vi "ServoAction.vi"(7 "face_dir":dbl(ring) items=["up"=0.1095, "up_up"=0.114637, "down"=0.073446, "back"=0.037435, "back_back"=0.035], 8 "Error In":errorcluster) -> (0 "Error Out":errorcluster)   [LabVIEW 2019]
uses:
  WSCbot_V3_Toolkit.lvlibp/WSCBOTV3_Toolkit/IO/LowLevel/IO_Chanel_DIO.ctl
  WSCbot_V3_Toolkit.lvlibp
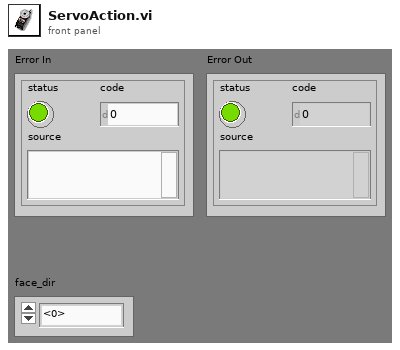
[diagram p1: front panel]
types:
  T1 = typedef "WSCbot_V3_Toolkit.lvlibp/IO_Chanel_DIO.ctl" = enum16{"A/DIO9", "A/DIO10", "C/DIO0", "C/DIO1", "C/DIO2", "C/DIO3", "C/DIO4", "C/DIO5", "C/DIO6"}
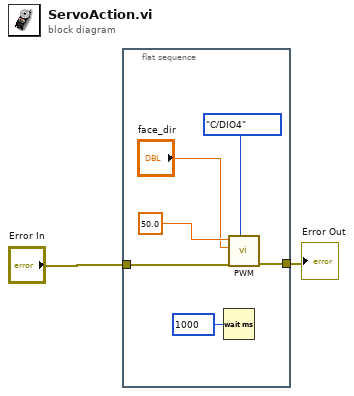
[diagram p0: block diagram]
diagram:
  n1 = flat-sequence {
    tunnel: "Error In" -> [w5]
    tunnel: [w4] -> w1
    frame #0 {
      n2 = Wait (ms)(milliseconds to wait=u32 1000) -> ()  [unwired: 1 out]
      n3 = call "PWM.vi"("IO_Chanel"=IO_Chanel_DIO."C/DIO4", "error in"=w5, "DutyCycle"="face_dir", "Frequency(Hz)"=50.0) -> ("error out"=w4:errorcluster)  [unwired: 7 in]
    }
  }
  "Error Out" <- w1
